vi "DLP_CalibrationPrints_XML_Read.vi"(8 "error in (no error)":errorcluster, 11 "Recipe XML File Path":path) -> (0 "error out":errorcluster, 2 "CalibrationPrints":T1)   [LabVIEW 2022 SP3]
uses:
  Controls/DLPConfig_CalibrationPrints.ctl
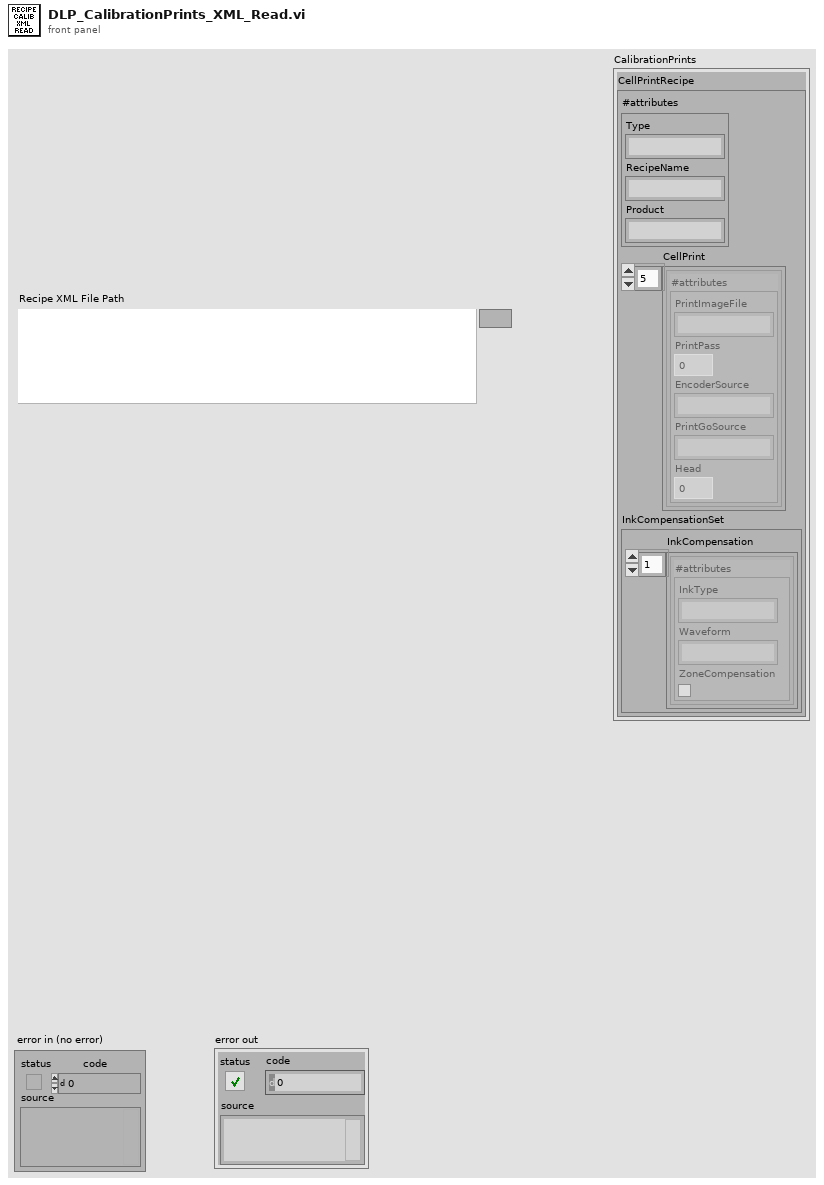
[diagram p1: front panel]
types:
  T1 = typedef "DLPConfig_CalibrationPrints.ctl" = cluster{"CellPrintRecipe":cluster{"#attributes":cluster{"Type":string, "RecipeName":string, "Product":string}, "CellPrint":cluster{"#attributes":cluster{"PrintImageFile":string, "PrintPass":i32, "EncoderSource":string, "PrintGoSource":string, "Head":i32}}[], "InkCompensationSet":cluster{"InkCompensation":cluster{"#attributes":cluster{"InkType":string, "Waveform":string, "ZoneCompensation":bool}}[]}}}
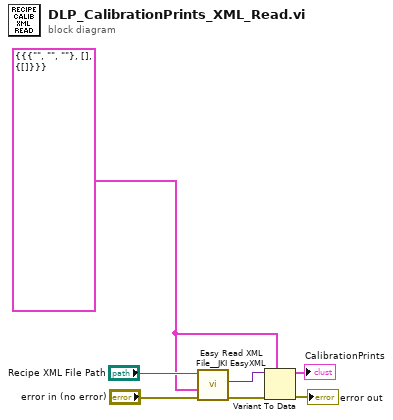
[diagram p0: block diagram]
diagram:
  w2 = T1 {"CellPrintRecipe"={"#attributes"={"Type"="", "RecipeName"="", "Product"=""}, "CellPrint"=[], "InkCompensationSet"={"InkCompensation"=[]}}} ("DLPRecipe")
  n1 = call <vilib>:"Easy Read XML File__JKI EasyXML.vi"("error in (no error)"="error in (no error)", "LabVIEW Data (Type)"=w2, "XML File Path"="Recipe XML File Path") -> ("error out"=w4:errorcluster, "LabVIEW Data"=w5:variant)  [unwired: 6 in, 1 out]
  n2 = Variant To Data(error in=w4, type=w2, Variant=w5) -> (data=→"CalibrationPrints":T1, error out=→"error out":errorcluster)
